vi "Lab1_A1.vi"() -> ()   [LabVIEW 2020]
panel:
  out "Multiplication":dbl
  out "Division":dbl
  out "Subtraction":dbl
  out "Addition":dbl
  in  "Variable 2":dbl
  in  "Variable 1":dbl
  in  "stop":bool
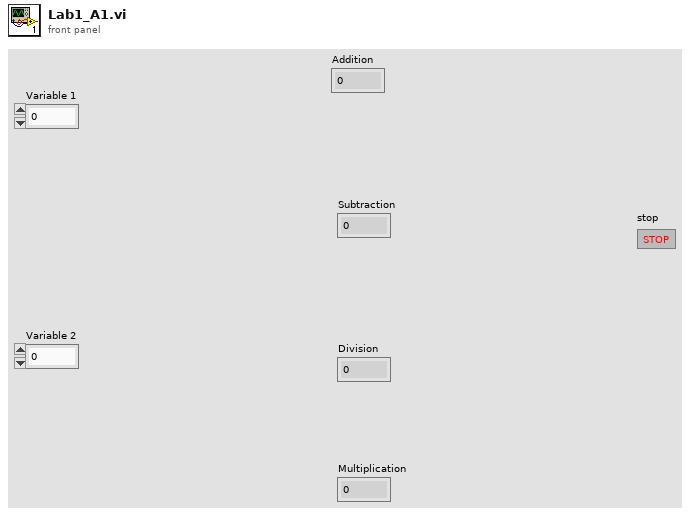
[diagram p1: front panel]
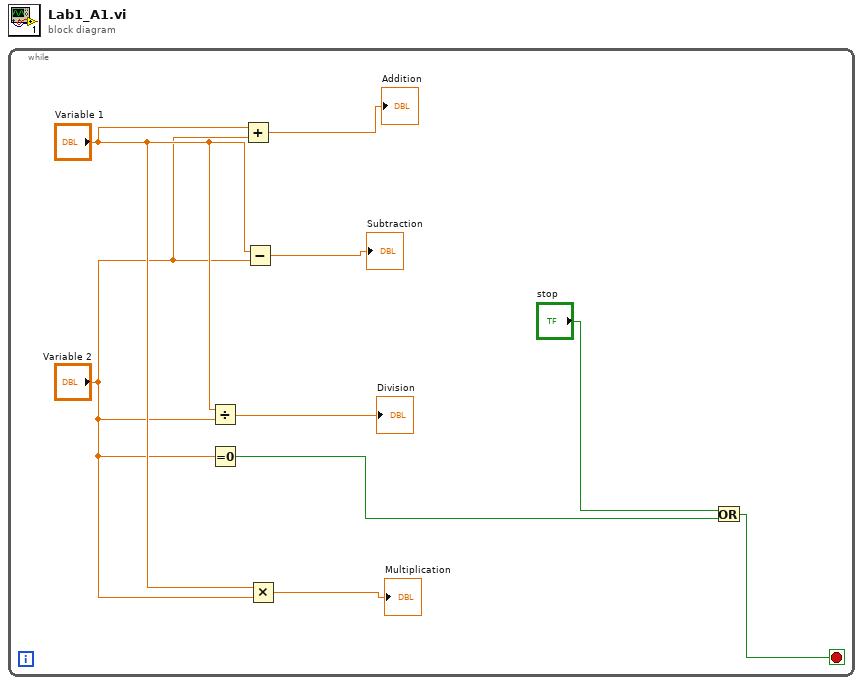
[diagram p0: block diagram]
diagram:
  n1 = while {
    stop <- w3 stop-if-true
    n2 = Divide(x="Variable 1", y="Variable 2") -> (x/y=→"Division":dbl)
    n3 = Equal To 0?(x="Variable 2") -> (x = 0?=w1:bool)
    n4 = Add(x="Variable 1", y="Variable 2") -> (x+y=→"Addition":dbl)
    n5 = Subtract(x="Variable 1", y="Variable 2") -> (x-y=→"Subtraction":dbl)
    n6 = Multiply(x="Variable 1", y="Variable 2") -> (x*y=→"Multiplication":dbl)
    n7 = Or(x="stop", y=w1) -> (x .or. y?=w3:bool)
  }
